vi "Read Scrubbers.vi"(8 "error in":errorcluster, 11 "Multi Scrubber in":refnum<class "Multi Scrubber.lvclass">) -> (0 "error out":errorcluster, 2 "Scrubbers":refnum<class "Scrubber.lvclass">[](array[class]), 3 "Multi Scrubber out":refnum<class "Multi Scrubber.lvclass">)   [LabVIEW 2020, in "Approval Tests.lvlib" / "Multi Scrubber.lvclass"]
uses:
  Multi Scrubber.lvclass
  Scrubber/Scrubber.lvclass
  Multi Scrubber.lvclass/Multi Scrubber.ctl
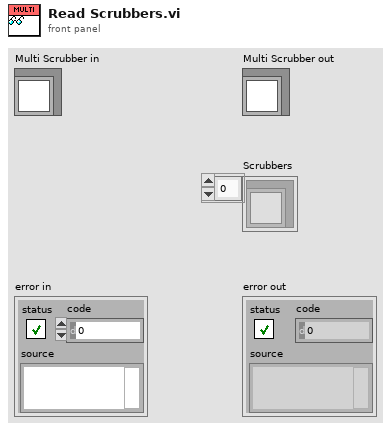
[diagram p1: front panel]
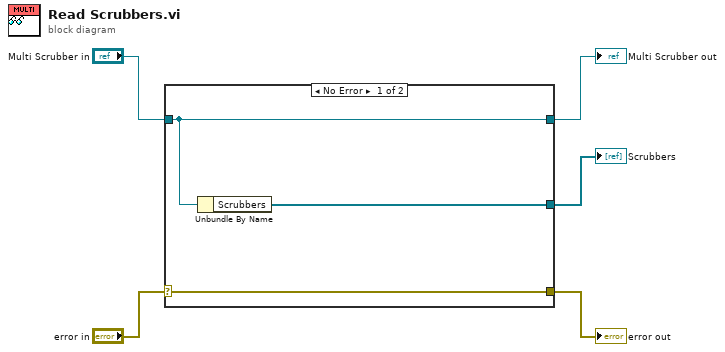
[diagram p0: block diagram]
diagram:
  n1 = case shown="No Error" "error in" {
    selector: "error in" -> [w8 w10]
    tunnel: [w8 w10] -> w4
    tunnel: [w7 w9] -> w2
    tunnel: "Multi Scrubber in" -> [w7 w9]
    tunnel: [w6 _] -> w1
    frame No Error {
      n2 = Unbundle By Name(w7) -> ("Scrubbers"=w6:refnum<class "Scrubber.lvclass">[])
    }
    frame Error {
    }
  }
  "error out" <- w4
  "Multi Scrubber out" <- w2
  "Scrubbers" <- w1
